vi "take_data (SubVI).vi"(8 "instrument in":T3, 11 "channel_settings":T2) -> (0 "instrument out":T3, 3 "Actual Sample Rate":dbl=10000.0 format="%0.2f", 5 "data_cluster":T1)   [LabVIEW 2022 SP3]
uses:
  <vilib>/DAQmx/configure/trigger.llb/DAQmx Start Trigger (Digital Edge).vi
  <vilib>/DAQmx/create/channels.llb/DAQmx Create Channel (AI-Voltage-Basic).vi
  <vilib>/DAQmx/configure/timing.llb/DAQmx Timing (Sample Clock).vi
  <resource>/objmgr/daqmx.rc
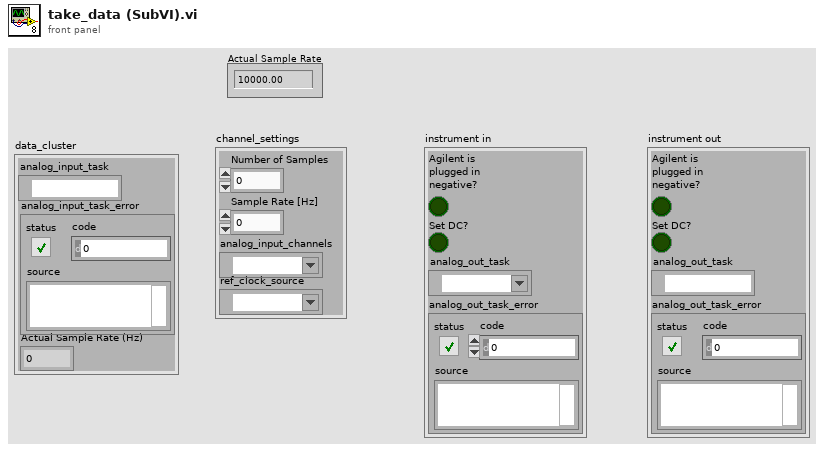
[diagram p1: front panel]
types:
  T1 = cluster{"analog_input_task":refnum<k21>, "analog_input_task_error":errorcluster, "Actual Sample Rate (Hz)":dbl}
  T2 = cluster{"Number of Samples":i32, "Sample Rate [Hz]":dbl, "analog_input_channels":tag, "ref_clock_source":tag}
  T3 = cluster{"Agilent is \nplugged in \nnegative?":bool, "Set DC?":bool, "analog_out_task":refnum<k21>, "analog_out_task_error":errorcluster}
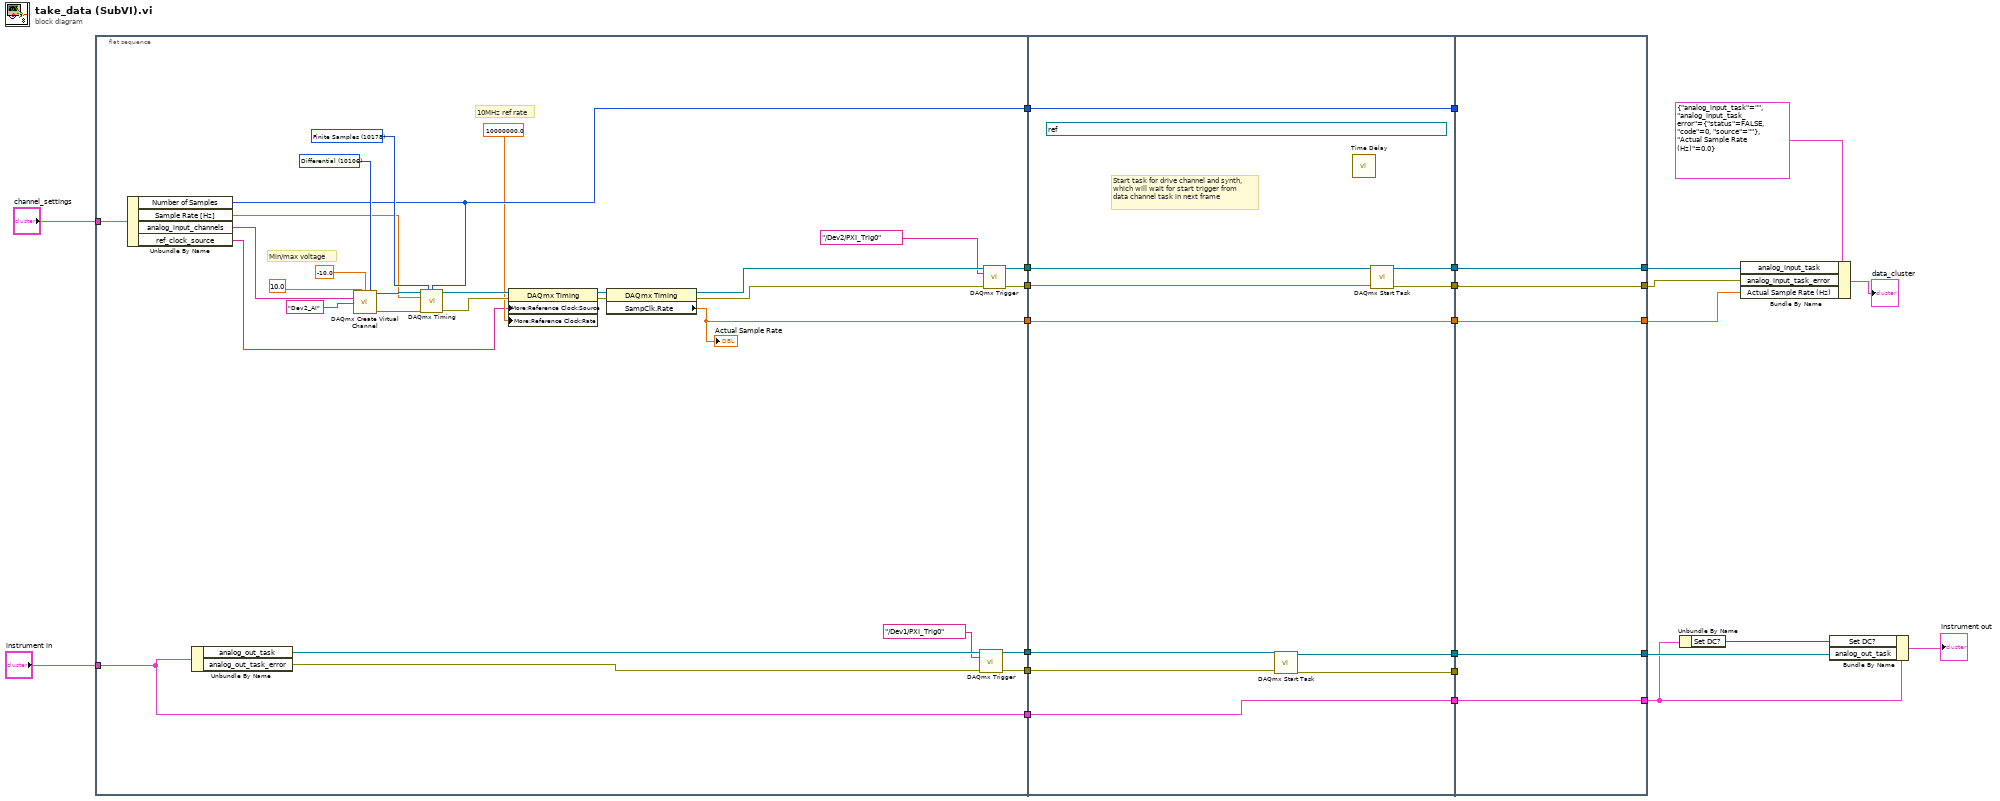
[diagram p0: block diagram]
diagram:
  n1 = flat-sequence {
    tunnel: [w34] -> w25
    tunnel: [w33] -> w24
    tunnel: [w47] -> w21
    tunnel: [w46] -> w20
    tunnel: [w26] -> w18
    tunnel: [w37] -> w15
    tunnel: [w36] -> w12
    tunnel: "channel_settings" -> [w44]
    tunnel: "instrument in" -> [w26]
    tunnel: w25 -> [w58]
    tunnel: w24 -> [w57]
    tunnel: [w56] -> w23
    tunnel: [w55] -> w22
    tunnel: w21 -> [w65]
    tunnel: w20 -> [w64]
    tunnel: [w63] -> w19
    tunnel: w18 -> [w63]
    tunnel: [w62] -> w17
    tunnel: [w61] -> w16
    tunnel: w15 -> [w60]
    tunnel: [w60] -> w14
    tunnel: [w59] -> w13
    tunnel: w12 -> [w59]
    tunnel: w23 -> [w67]
    tunnel: w22 -> [w66]
    tunnel: w19 -> [w70]
    tunnel: w17 -> [w69]
    tunnel: w16 -> [_]
    tunnel: w14 -> [_]
    tunnel: w13 -> [w68]
    tunnel: [w67] -> w3
    tunnel: [w66] -> w2
    tunnel: [w70] -> w8
    tunnel: [w69] -> w10
    tunnel: [w68] -> w1
    frame #0 {
      w48 = 10106 items=["default"=-1, "RSE"=10083, "NRSE"=10078, "Differential"=10106, "Pseudodifferential"=12529] ("input terminal configuration")
      w45 = 10178 items=["Finite Samples"=10178, "Continuous Samples"=10123, "Hardware Timed Single Point"=12522] ("sample mode")
      # "10MHz ref rate"
      # "Min/max voltage"
      n2 = Unbundle By Name(w44) -> ("Number of Samples"=w37:i32, "Sample Rate [Hz]"=w38:dbl, "analog_input_channels"=w43:tag, "ref_clock_source"=w27:tag)
      n3 = Unbundle By Name(w26) -> ("analog_out_task"=w42:refnum<k21>, "analog_out_task_error"=w41:errorcluster)
      n4 = call-poly <vilib>:"DAQmx Create Virtual Channel.vi"("maximum value"=10.0, "minimum value"=-10.0, "input terminal configuration"=w48, "physical channels"=w43, "name to assign"="Dev2_AI") -> ("task out"=w49:refnum<k21>, "error out"=w50:errorcluster)  [unwired: 9 in]
      n5 = call-poly <vilib>:"DAQmx Timing.vi"("task/channels in"=w49, "sample mode"=w45, "samples per channel"=w37, "rate"=w38, "error in"=w50) -> ("task out"=w51:refnum<k21>, "error out"=w52:errorcluster)  [unwired: 9 in]
      n6 = property class="DAQmx Timing"(reference=w51, error in=w52, "More:Reference Clock:Source"=w27, "More:Reference Clock:Rate"=10000000.0 ("RefClk.Rate")) -> (reference out=w53:refnum<k21>, error out=w54:errorcluster)
      n7 = property class="DAQmx Timing"(reference=w53, error in=w54) -> (reference out=w32:refnum<k21>, error out=w31:errorcluster, "SampClk.Rate"=w36:dbl)
      "Actual Sample Rate" <- w36
      n8 = call-poly <vilib>:"DAQmx Trigger.vi"("task/channels in"=w42, "source"=tag "/Dev1/PXI_Trig0", "error in"=w41) -> ("task out"=w47:refnum<k21>, "error out"=w46:errorcluster)  [unwired: 11 in]
      n9 = call-poly <vilib>:"DAQmx Trigger.vi"("task/channels in"=w32, "source"=tag "/Dev2/PXI_Trig0", "error in"=w31) -> ("task out"=w34:refnum<k21>, "error out"=w33:errorcluster)  [unwired: 11 in]
    }
    frame #1 {
      (unwired) refnum<k21> "Dev2/ai0:7, Dev2/ai23, Dev2/ai21, Dev2/ai19, Dev2/ai17, Dev2/ai16, Dev2/ai22, Dev2/ai20, Dev2/ai18" ("ChannelsToRead")
      # "Start task for drive channel and synth,\nwhich will wait for start trigger from \ndata channel task in next frame"
      n10 = call <vilib>:"DAQmx Start Task.vi"("task/channels in"=w65, "error in"=w64) -> ("task out"=w62:refnum<k21>, "error out"=w61:errorcluster)  [unwired: 12 in]
      n11 = call "Time Delay"() -> ()  [unwired: 11 in, 1 out]
      n12 = call <vilib>:"DAQmx Start Task.vi"("task/channels in"=w58, "error in"=w57) -> ("task out"=w56:refnum<k21>, "error out"=w55:errorcluster)  [unwired: 12 in]
    }
    frame #2 {
    }
  }
  n13 = Unbundle By Name(w8) -> ("Set DC?"=w7:bool)
  n14 = Bundle By Name(cluster=T1 {"analog_input_task"="", "analog_input_task_error"={"status"=FALSE, "code"=0, "source"=""}, "Actual Sample Rate (Hz)"=0.0} ("input cluster"), "analog_input_task"=w3, "analog_input_task_error"=w2, "Actual Sample Rate (Hz)"=w1) -> (→"data_cluster":T1)
  n15 = Bundle By Name(cluster=w8, "Set DC?"=w7, "analog_out_task"=w10) -> (→"instrument out":T3)
